vi "CANFD Set Filter.vi"(7 "Len":u8, 8 "error in (no error)":errorcluster, 9 "pCanFilter":T1, 10 "CANIndex":u8, 11 "DevHandle":i32) -> (0 "error out":errorcluster, 1 "pCanFilter out":T1, 3 "function return":i32)   [LabVIEW 2010, in "usb2canfd.lvlib"]
doc: "int WINAPI CANFD_SetFilter(int DevHandle, unsigned char CANIndex, CANFD_FILTER_CONFIG *pCanFilter,unsigned char Len);"
uses:
  usb2canfd.lvlib
  examples/Labview/PublicFiles/USB2XXX.dll
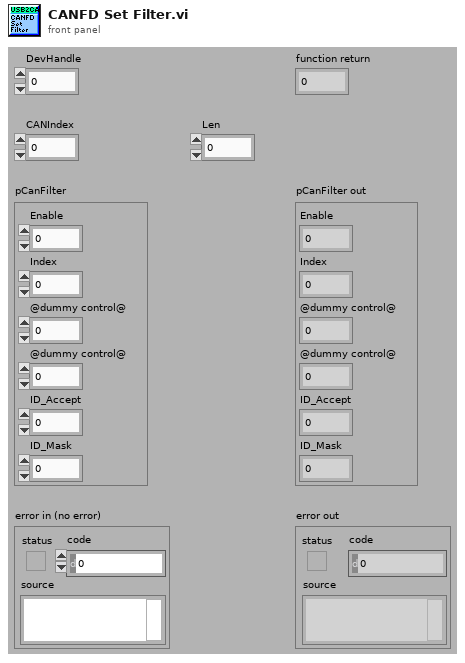
[diagram p1: front panel]
types:
  T1 = cluster{"Enable":u8, "Index":u8, "@dummy control@":i8, "@dummy control@":i8, "ID_Accept":u32, "ID_Mask":u32}
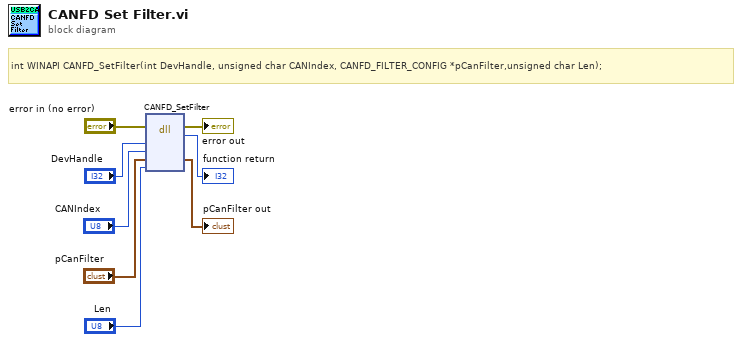
[diagram p0: block diagram]
diagram:
  # "int WINAPI CANFD_SetFilter(int DevHandle, unsigned char CANIndex, CANFD_FILTER_CONFIG *pCanFilter,unsigned char Len);"
  n1 = dll-call lib="E:/OtherWork/STM32/USB2XXX_Example/examples/Labview/PublicFiles/USB2XXX.*" fn="CANFD_SetFilter"(error in="error in (no error)", "DevHandle"="DevHandle", "CANIndex"="CANIndex", "pCanFilter"="pCanFilter", "Len"="Len") -> (error out=→"error out":errorcluster, →"function return":i32, "pCanFilter"=→"pCanFilter out":T1)  [unwired: 5 in, 1 out]
